vi "JSON-ProcessDBData.vi"(7 "JSON string":string, 8 "error in (no error)":errorcluster) -> (0 "error out":errorcluster, 3 "Update Inventory Cluster":T1)   [LabVIEW 2013]
uses:
  <userlib>/_OpenG.lib/array/array.llb/Reorder 1D Array2 (String)__ogtk.vi
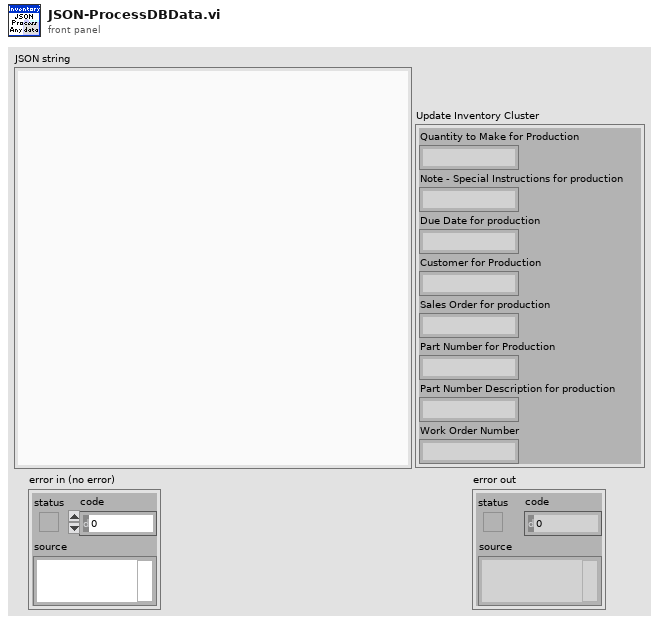
[diagram p1: front panel]
types:
  T1 = cluster{"Quantity to Make for Production":string, "Note - Special Instructions for production":string, "Due Date for production":string, "Customer for Production":string, "Sales Order for production":string, "Part Number for Production":string, "Part Number Description for production":string, "Work Order Number":string}
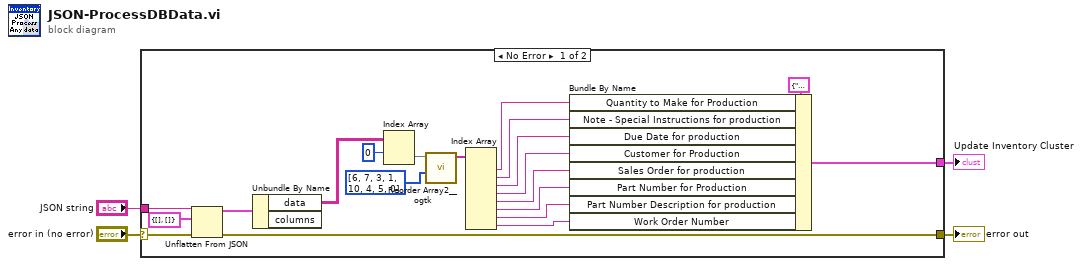
[diagram p0: block diagram]
diagram:
  n1 = case shown="No Error" "error in (no error)" {
    selector: "error in (no error)" -> [w24 w25]
    tunnel: [w5 w25] -> w3
    tunnel: "JSON string" -> [w23 _]
    tunnel: [w6 _] -> w1
    frame No Error {
      n2 = Unflatten From JSON(JSON string=w23, type and defaults=cluster{"data":string[][], "columns":string[]} {"data"=[], "columns"=[]}, error in (no error)=w24) -> (value=w22:cluster{"data":string[][], "columns":string[]}, error out=w5:errorcluster)  [unwired: 4 in]
      n3 = Unbundle By Name(w22) -> ("data"=w19:string[][])  [unwired: 1 out]
      n4 = Index Array(array=w19, index (row)=0) -> (element=w17:string[])  [unwired: 1 in]
      n5 = call-poly <userlib>:"Reorder Array2__ogtk.vi"("indices"=i32[] [6, 7, 3, 1, 10, 4, 5, 0], "array"=w17) -> ("reordered array"=w15:string[])  [unwired: 9 in]
      n6 = Index Array(array=w15) -> (element #1=w14:string, element #2=w13:string, element #3=w12:string, element #4=w11:string, element #5=w10:string, element #6=w9:string, element #7=w8:string, element #8=w7:string)  [unwired: 8 in]
      n7 = Bundle By Name(cluster=T1 {"Quantity to Make for Production"="", "Note - Special Instructions for production"="", "Due Date for production"="", "Customer for Production"="", "Sales Order for production"="", "Part Number for Production"="", "Part Number Description for production"="", "Work Order Number"=""} ("Cluster for Inventory 2"), "Quantity to Make for Production"=w14, "Note - Special Instructions for production"=w13, "Due Date for production"=w12, "Customer for Production"=w11, "Sales Order for production"=w10, "Part Number for Production"=w9, "Part Number Description for production"=w8, "Work Order Number"=w7) -> (w6:T1)
    }
    frame Error {
    }
  }
  "error out" <- w3
  "Update Inventory Cluster" <- w1
